vi "Arinc Database Parser.vi"(7 "Database []":T1) -> (8 "String":string)   [LabVIEW 2017]
uses:
  Controls/Database_Array.ctl
  Controls/Encoding.ctl
  <userlib>/_OpenG.lib/array/array.llb/Remove Duplicates from 1D Array (I32)__ogtk.vi
  <userlib>/_OpenG.lib/array/array.llb/Filter 1D Array with Scalar (I32)__ogtk.vi
  <userlib>/_OpenG.lib/array/array.llb/Index 1D Array Elements (I32)__ogtk.vi
  <userlib>/_OpenG.lib/array/array.llb/Index 1D Array Elements (String)__ogtk.vi
  <userlib>/_OpenG.lib/array/array.llb/Remove Duplicates from 1D Array (String)__ogtk.vi
  <userlib>/_OpenG.lib/array/array.llb/Index 1D Array Elements (DBL)__ogtk.vi
panel:
  out "Label Rate":i32
  out "Parameters":string[](array[string])
  out "Label Name and Rate Same?":bool
  out "Channel Name and Rate Same?":bool
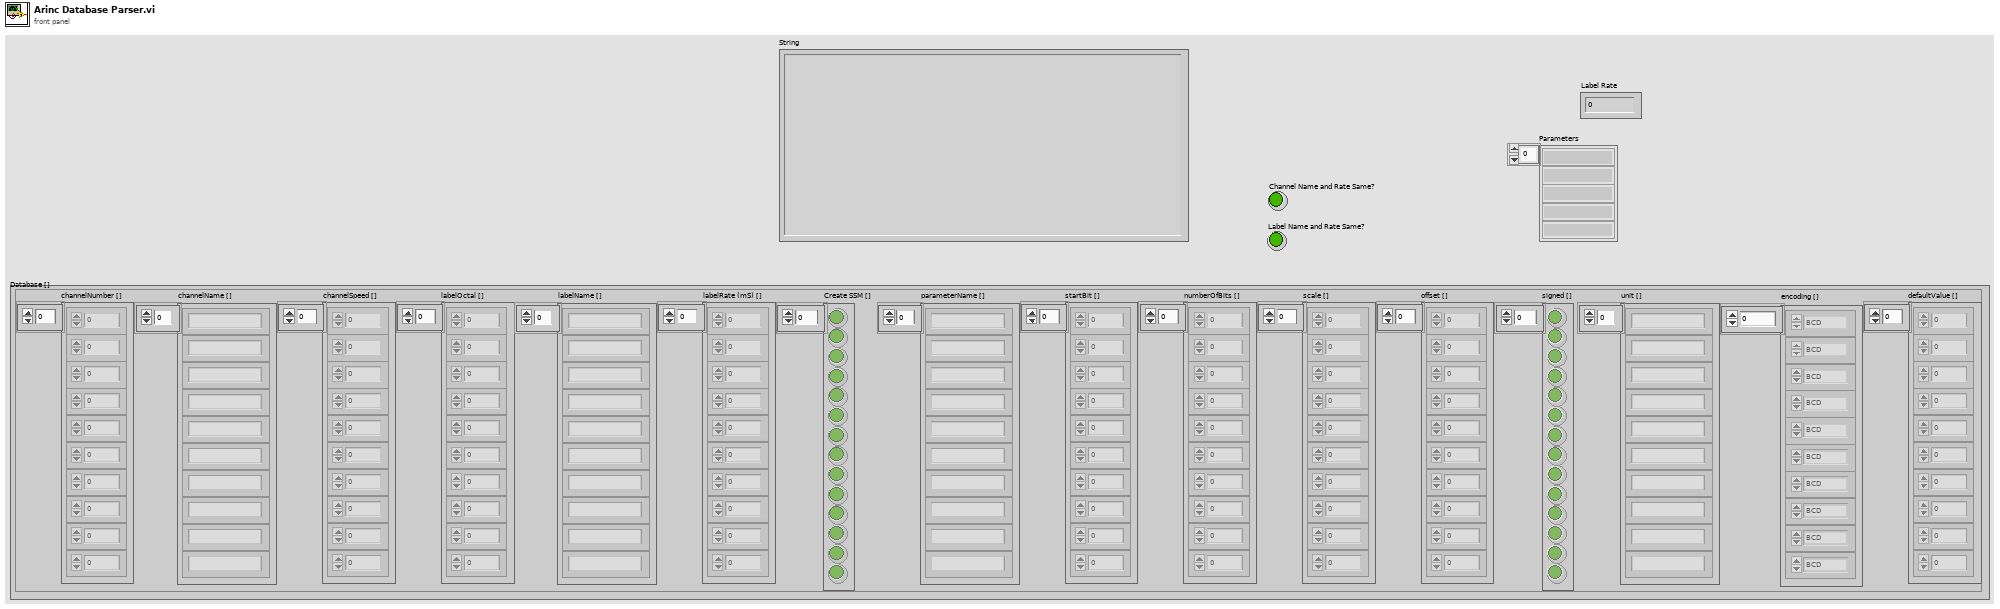
[diagram p1: front panel]
types:
  T1 = typedef "Database_Array.ctl" = cluster{"channelNumber []":i32[], "channelName []":string[], "channelSpeed []":i32[], "labelOctal []":i32[], "labelName []":string[], "labelRate (mS) []":i32[], "Create SSM []":bool[], "parameterName []":string[], "startBit []":i32[], "numberOfBits []":i32[], "scale []":dbl[], "offset []":dbl[], "signed []":bool[], "unit []":string[], "encoding []":T2[], "defaultValue []":dbl[]}
  T2 = typedef "Encoding.ctl" = enum16{"BCD", "BNR", "Discrete"}
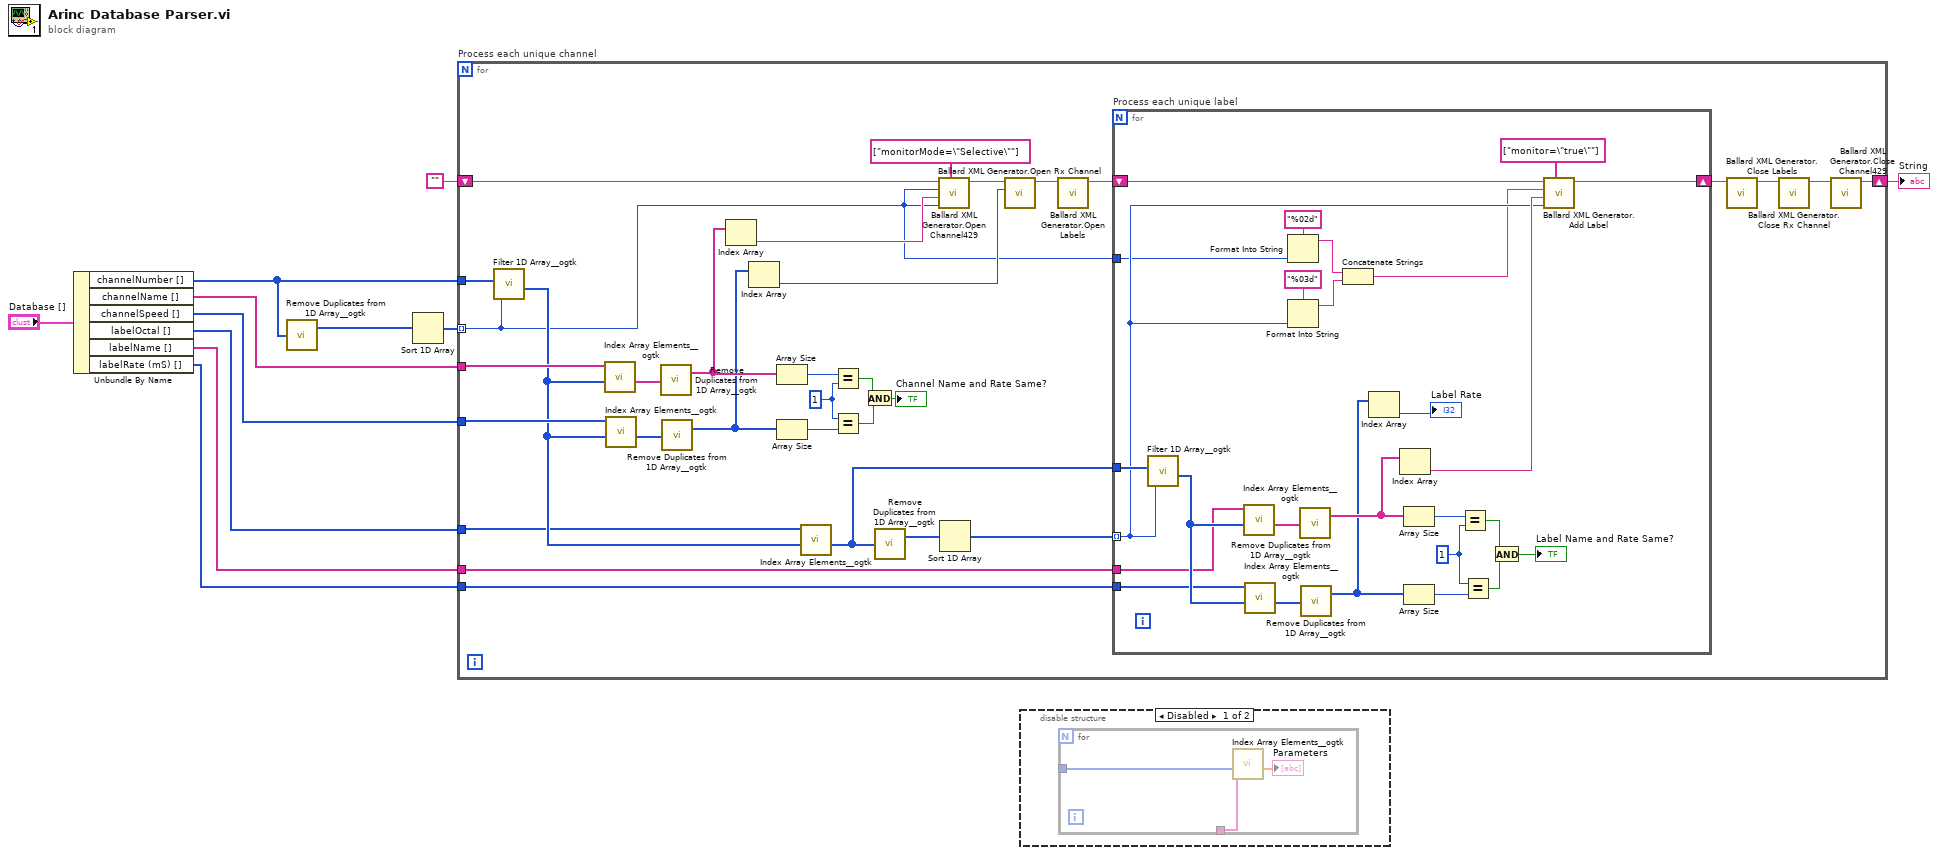
[diagram p0: block diagram]
diagram:
  n1 = Unbundle By Name("Database []") -> ("channelNumber []"=w6:i32[], "channelName []"=w5:string[], "channelSpeed []"=w4:i32[], "labelOctal []"=w3:i32[], "labelName []"=w2:string[], "labelRate (mS) []"=w1:i32[])
  n2 = call-poly <userlib>:"Remove Duplicates from 1D Array__ogtk.vi"("Input Array"=w6) -> ("Output Array"=w10:i32[])  [unwired: 1 out]
  n3 = Sort 1D Array(array=w10) -> (sorted array=w11:i32[])
  n4 = for "Process each unique channel" {
    tunnel: w11 -> [w12] mode=indexing
    tunnel: w6 -> [w43]
    tunnel: w5 -> [w42]
    tunnel: w4 -> [w39]
    tunnel: w3 -> [w31]
    shift-right: [w15] -> w8
    shift-left: "" -> [w24]
    tunnel: w2 -> [w14]
    tunnel: w1 -> [w13]
    w36 = 1 ("size(s)")
    n5 = call-poly <userlib>:"Filter 1D Array__ogtk.vi"("items to filter"=w12, "array"=w43) -> ("filtered item indices"=w32:i32[])  [unwired: 4 in, 1 out]
    n6 = call-poly <userlib>:"Index Array Elements__ogtk.vi"("indices"=w32, "array"=w42) -> ("elements"=w41:string[])  [unwired: 9 in]
    n7 = call-poly <userlib>:"Index Array Elements__ogtk.vi"("indices"=w32, "array"=w39) -> ("elements"=w40:i32[])  [unwired: 9 in]
    n8 = call-poly <userlib>:"Remove Duplicates from 1D Array__ogtk.vi"("Input Array"=w41) -> ("Output Array"=w27:string[])  [unwired: 1 out]
    n9 = call-poly <userlib>:"Remove Duplicates from 1D Array__ogtk.vi"("Input Array"=w40) -> ("Output Array"=w26:i32[])  [unwired: 1 out]
    n10 = Index Array(array=w27) -> (element=w25:string)  [unwired: 1 in]
    n11 = Index Array(array=w26) -> (element=w20:i32)  [unwired: 1 in]
    n12 = Array Size(array=w27) -> (size(s)=w38:i32)
    n13 = Array Size(array=w26) -> (size(s)=w37:i32)
    n14 = call-poly <userlib>:"Index Array Elements__ogtk.vi"("indices"=w32, "array"=w31) -> ("elements"=w28:i32[])  [unwired: 9 in]
    n15 = Equal?(x=w38, y=w36) -> (x = y?=w35:bool)
    n16 = Equal?(x=w36, y=w37) -> (x = y?=w34:bool)
    n17 = And(x=w35, y=w34) -> (x .and. y?=→"Channel Name and Rate Same?":bool)
    n18 = call-poly <userlib>:"Remove Duplicates from 1D Array__ogtk.vi"("Input Array"=w28) -> ("Output Array"=w30:i32[])  [unwired: 1 out]
    n19 = call "Ballard XML Generator.Open Channel429.vi"("other params"=string[] ["monitorMode=\"Selective\""], "hardware channel"=w12, "name"=w25, "id"=w12, "string in"=w24) -> ("string out"=w21:string)  [unwired: 6 in]
    n20 = Sort 1D Array(array=w30) -> (sorted array=w29:i32[])
    n21 = call "Ballard XML Generator.Open Rx Channel.vi"("speedKHz"=w20, "string in"=w21) -> ("string out"=w22:string)  [unwired: 9 in]
    n22 = call "Ballard XML Generator.Open Labels.vi"("string in"=w22) -> ("string out"=w19:string)  [unwired: 10 in]
    n23 = for "Process each unique label" {
      tunnel: w29 -> [w48] mode=indexing
      tunnel: w28 -> [w69]
      shift-right: [w54] -> w18
      shift-left: w19 -> [w55]
      tunnel: w14 -> [w52]
      tunnel: w13 -> [w51]
      tunnel: w12 -> [w47]
      w64 = 1 ("size(s)")
      n24 = call-poly <userlib>:"Filter 1D Array__ogtk.vi"("items to filter"=w48, "array"=w69) -> ("filtered item indices"=w57:i32[])  [unwired: 4 in, 1 out]
      n25 = call-poly <userlib>:"Index Array Elements__ogtk.vi"("indices"=w57, "array"=w52) -> ("elements"=w68:string[])  [unwired: 9 in]
      n26 = call-poly <userlib>:"Index Array Elements__ogtk.vi"("indices"=w57, "array"=w51) -> ("elements"=w67:i32[])  [unwired: 9 in]
      n27 = Format Into String(format string="%02d", w47) -> (resulting string=w46:string)  [unwired: 2 in, 1 out]
      n28 = Format Into String(format string="%03d", w48) -> (resulting string=w45:string)  [unwired: 2 in, 1 out]
      n29 = call-poly <userlib>:"Remove Duplicates from 1D Array__ogtk.vi"("Input Array"=w68) -> ("Output Array"=w60:string[])  [unwired: 1 out]
      n30 = call-poly <userlib>:"Remove Duplicates from 1D Array__ogtk.vi"("Input Array"=w67) -> ("Output Array"=w59:i32[])  [unwired: 1 out]
      n31 = Concatenate Strings(w46, w45) -> (w44:string)
      n32 = Index Array(array=w59) -> (element=→"Label Rate":i32)  [unwired: 1 in]
      n33 = Index Array(array=w60) -> (element=w53:string)  [unwired: 1 in]
      n34 = Array Size(array=w60) -> (size(s)=w66:i32)
      n35 = Array Size(array=w59) -> (size(s)=w65:i32)
      n36 = Equal?(x=w66, y=w64) -> (x = y?=w63:bool)
      n37 = Equal?(x=w64, y=w65) -> (x = y?=w62:bool)
      n38 = And(x=w63, y=w62) -> (x .and. y?=→"Label Name and Rate Same?":bool)
      n39 = call "Ballard XML Generator.Add Label.vi"("other params"=string[] ["monitor=\"true\""], "label decimal"=w48, "name"=w53, "id"=w44, "string in"=w55) -> ("string out"=w54:string)  [unwired: 6 in]
    }
    n40 = call "Ballard XML Generator.Close Labels.vi"("string in"=w18) -> ("string out"=w17:string)  [unwired: 10 in]
    n41 = call "Ballard XML Generator.Close Rx Channel.vi"("string in"=w17) -> ("string out"=w16:string)  [unwired: 10 in]
    n42 = call "Ballard XML Generator.Close Channel429.vi"("string in"=w16) -> ("string out"=w15:string)  [unwired: 10 in]
  }
  "String" <- w8
  n43 = disable-structure shown="Disabled" {
    frame Disabled {
      n44 = for {
        tunnel: _ -> [w71]
        tunnel: _ -> [w72]
        n45 = call-poly <userlib>:"Index Array Elements__ogtk.vi"("indices"=w71, "array"=w72) -> ("elements"=→"Parameters":dbl[])  [unwired: 9 in]
      }
    }
    frame Enabled {
    }
  }
